vi "TW Adjust lib ICON.vi"(6 "Debug":bool, 7 "Overlay Icon":refnum<class "Icon.lvclass">, 8 "error in":errorcluster, 10 "Library Name":string="TemplatePlugin.lvclass", 11 "Name to Lib Map":map{string, refnum<vi>}(c390)) -> (0 "error out":errorcluster caption="error in", 3 "Name to Lib Map out":map{string, refnum<vi>}(c390), 4 "Result for debugging":cluster{"Name":string, picture[]}[](array[cluster]))   [LabVIEW 2021, in "Plugin Generator.lvlib"]
uses:
  Plugin Generator.lvlib
  <vilib>/LabVIEW Icon API/lv_icon/Classes/Icon/Icon.lvclass
  <vilib>/LabVIEW Icon API/Support/Get Data from Icon Class.vi
  <vilib>/LabVIEW Icon API/lv_icon/Classes/Layer/Substitute Layer.vi
  <vilib>/LabVIEW Icon API/Support/Get Icon Class from Data.vi
  <vilib>/LabVIEW Icon API/Set VI Icon.vi
  <vilib>/LabVIEW Icon API/LabVIEW Icon API.lvlib
  <vilib>/LabVIEW Icon API/Set Text Icon/Text-Based VI Icon.lvlib
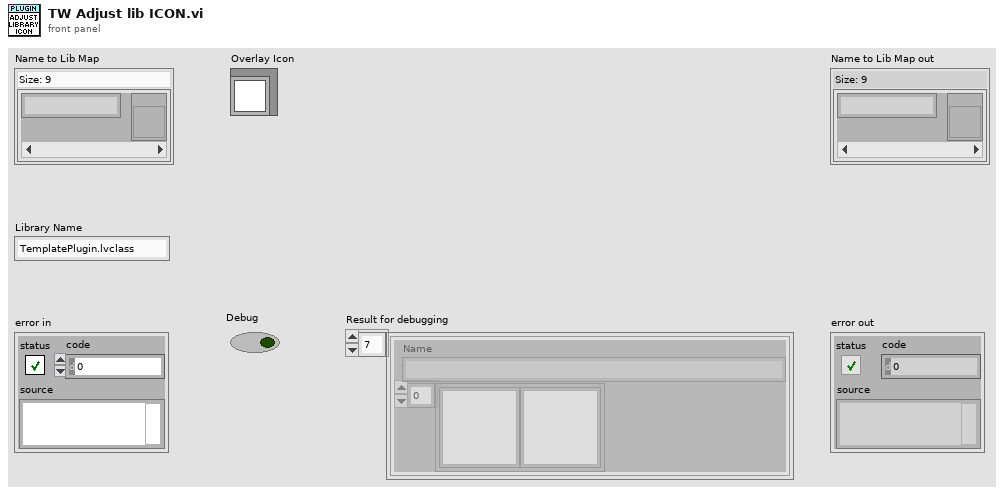
[diagram p1: front panel]
types:
  T1 = typedef "imagedata.ctl" = cluster{"image type":i32, "image depth":i32, "image":u8[], "mask":u8[], "colors":u32[], "Rectangle":cluster{"left":i16, "top":i16, "right":i16, "bottom":i16}}
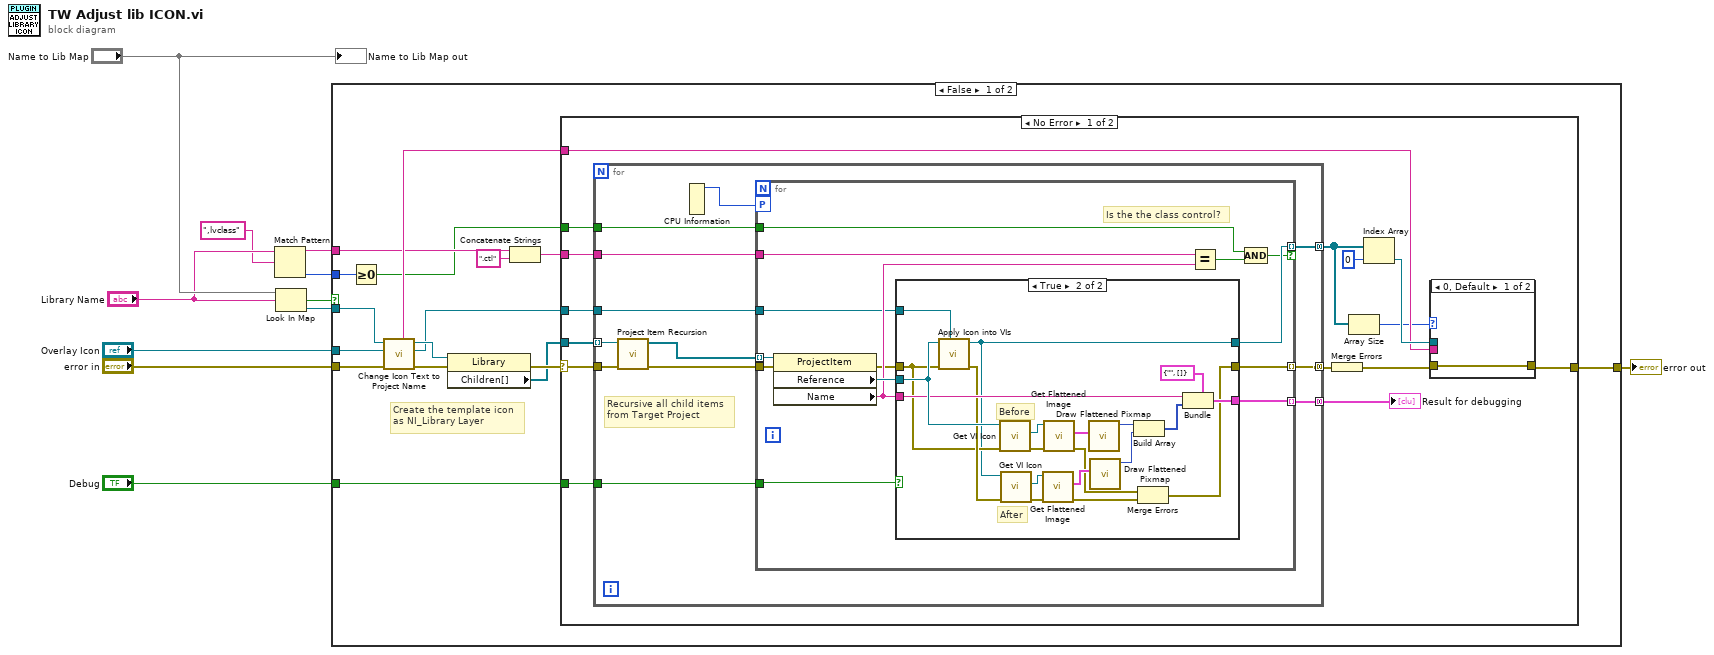
[diagram p0: block diagram]
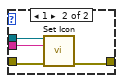
[diagram p2: hidden frame]
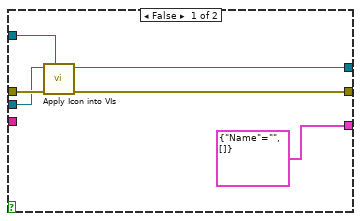
[diagram p3: hidden frame]
diagram:
  n1 = Match Pattern(string="Library Name", regular expression=",lvclass") -> (before substring=w1:string, offset past match=w2:i32)  [unwired: 1 in, 2 out]
  n2 = Look In Map(map="Name to Lib Map", key="Library Name") -> (key not found?=w10:bool, value=w9:refnum<vi>)  [unwired: 1 in]
  n3 = case shown="False" w10 {
    tunnel: w9 -> [w27 _]
    tunnel: "Debug" -> [w24 _]
    tunnel: "error in" -> [w23 w101]
    tunnel: [w22 w101] -> w6
    tunnel: "Overlay Icon" -> [w19 _]
    tunnel: w2 -> [w17 _]
    tunnel: w1 -> [w15 _]
    frame False {
      # "Create the template icon\nas NI_Library Layer"
      n4 = Greater Or Equal To 0?(x=w17) -> (x >= 0?=w12:bool)
      n5 = call "Change Icon Text to Project Name.vi"("error in"=w23, "Overlay Icon"=w19, "Lvclass Ref in"=w27) -> ("error out"=w26:errorcluster, "Layer.lvclass out"=w20:refnum<class "Layer.lvclass">, "Lvclass Ref out"=w21:refnum<vi>, "Body Text.Line 1 text"=w18:string)  [unwired: 5 in]
      n6 = property class="Library"(reference=w21, error in=w26) -> (error out=w25:errorcluster, "Children[]"=w16:refnum<vi>[])  [unwired: 1 out]
      n7 = Concatenate Strings(w15, ".ctl" ("string")) -> (w13:string)
      n8 = case shown="No Error" w25 {
        selector: w25 -> [w32 w100]
        tunnel: w16 -> [w42 _]
        tunnel: w20 -> [w40 _]
        tunnel: w24 -> [w39 _]
        tunnel: [w34 w100] -> w22
        tunnel: w18 -> [w33 _]
        tunnel: w13 -> [w31 _]
        tunnel: w12 -> [w30 _]
        frame No Error {
          n9 = for {
            tunnel: w42 -> [w59] mode=indexing
            tunnel: [w57] -> w41 mode=concatenating
            tunnel: w40 -> [w55]
            tunnel: w39 -> [w54]
            tunnel: [w53] -> w29 mode=concatenating
            tunnel: [w52] -> w36 mode=concatenating
            tunnel: w32 -> [w51]
            tunnel: w31 -> [w50]
            tunnel: w30 -> [w49]
            # "Recursive all child items\nfrom Target Project"
            n10 = call "Project Item Recursion.vi"("error in"=w51, "TargetItem in"=w59) -> ("error out"=w56:errorcluster, "TargetItem out"=w58:refnum<vi>[])  [unwired: 8 in]
            n11 = CPU Information() -> (4:w48:i32)  [unwired: 3 out]
            n12 = for {
              tunnel: w58 -> [w73] mode=indexing
              tunnel: w56 -> [w72]
              tunnel: [w71] -> w57 mode=indexing
              tunnel: w55 -> [w65]
              workers-P: w48 -> [_]
              tunnel: w54 -> [w66]
              tunnel: [w64] -> w53 mode=indexing if=w61
              tunnel: [w68] -> w52 mode=indexing
              tunnel: w50 -> [w63]
              tunnel: w49 -> [w60]
              # "Is the the class control?"
              n13 = property class="ProjectItem"(reference=w73, error in=w72) -> (error out=w67:errorcluster, "Reference"=w70:refnum<vi>, "Name"=w69:string)  [unwired: 1 out]
              n14 = case shown="True" w66 {
                tunnel: [cluster{"Name":string, picture[]} {"Name"="", []} ("cluster") w99] -> w71
                tunnel: w70 -> [w74 w98]
                tunnel: w69 -> [_ w97]
                tunnel: [w77 w95] -> w68
                tunnel: w67 -> [w79 w82]
                tunnel: w65 -> [w78 w81]
                tunnel: [w75 w80] -> w64
                frame False {
                  n15 = call "Apply Icon into VIs.vi"("Substitute Layer"=w78, "error in"=w79, "VI in"=w74) -> ("error out"=w77:errorcluster, "VI Refnum out"=w75:refnum<vi>)  [unwired: 7 in]
                }
                frame True {
                  # "After"
                  # "Before"
                  n16 = call "Apply Icon into VIs.vi"("Substitute Layer"=w81, "error in"=w82, "VI in"=w98) -> ("error out"=w96:errorcluster, "VI Refnum out"=w80:refnum<vi>)  [unwired: 7 in]
                  n17 = call <vilib>:"Get VI Icon.vi"("error in (no error)"=w82, "VI Refnum in"=w98) -> ("error out"=w86:errorcluster, "Icon"=w92:refnum<class "Icon.lvclass">)  [unwired: 7 in, 1 out]
                  n18 = call <vilib>:"Get VI Icon.vi"("error in (no error)"=w96, "VI Refnum in"=w80) -> ("error out"=w85:errorcluster, "Icon"=w94:refnum<class "Icon.lvclass">)  [unwired: 7 in, 1 out]
                  n19 = call <vilib>:"Get Flattened Image.vi"("error in (no error)"=w85, "lv_icon.lvlib:Icon.lvclass in"=w94) -> ("error out"=w83:errorcluster, "Color Image"=w93:T1)  [unwired: 6 in, 2 out]
                  n20 = call <vilib>:"Get Flattened Image.vi"("error in (no error)"=w86, "lv_icon.lvlib:Icon.lvclass in"=w92) -> ("error out"=w84:errorcluster, "Color Image"=w91:T1)  [unwired: 6 in, 2 out]
                  n21 = call <vilib>:"Draw Flattened Pixmap.vi"("image data"=w91) -> ("new picture"=w90:picture)  [unwired: 8 in]
                  n22 = call <vilib>:"Draw Flattened Pixmap.vi"("image data"=w93) -> ("new picture"=w89:picture)  [unwired: 8 in]
                  n23 = Build Array(w90, w89) -> (w88:picture[])
                  n24 = Merge Errors(w84, w83) -> (w95:errorcluster)
                  n25 = Bundle(cluster=cluster{"Name":string, picture[]} {"Name"="", []}, "Name"=w97, w88) -> (w99:cluster{"Name":string, picture[]})
                }
              }
              n26 = Equal?(x=w63, y=w69) -> (x = y?=w62:bool)
              n27 = Compound Arithmetic op=AND(w60, w62) -> (w61:bool)
            }
          }
          "Result for debugging" <- w41
          n28 = Merge Errors(w36) -> (w35:errorcluster)
          n29 = Array Size(array=w29) -> (size(s)=w28:i32)
          n30 = Index Array(array=w29, index=0) -> (element=w37:refnum<vi>)
          n31 = case shown="0, Default" w28 {
            tunnel: w37 -> [_ w47]
            tunnel: w35 -> [w43 w46]
            tunnel: [w43 w45] -> w34
            tunnel: w33 -> [_ w44]
            frame 0, Default {
            }
            frame 1 {
              n32 = call <vilib>:"Set Icon.vi"("VI"=w47, "user-supplied text (\"\" - use VI file name)"=w44, "error in"=w46) -> ("error out"=w45:errorcluster)  [unwired: 11 in, 1 out]
            }
          }
        }
        frame Error {
        }
      }
    }
    frame True {
    }
  }
  "error out" <- w6
  "Name to Lib Map out" <- "Name to Lib Map"
